vi "ETL Initialize API Connection.vi"(8 "error in (no error)":errorcluster, 11 "Base URL":string) -> (0 "error out":errorcluster, 3 "REST Client out":refnum<class "REST Client.lvclass">)   [LabVIEW 2024, in "ETL API.lvlib"]
uses:
  ETL API.lvlib
  <vilib>/addons/_JKI.lib/REST Client/classes/REST Client/REST Client.lvclass
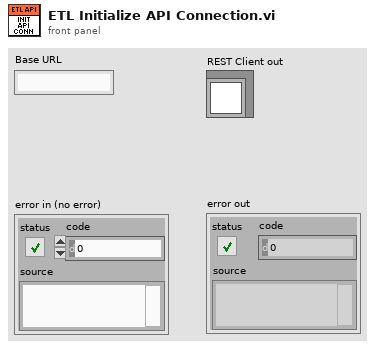
[diagram p1: front panel]
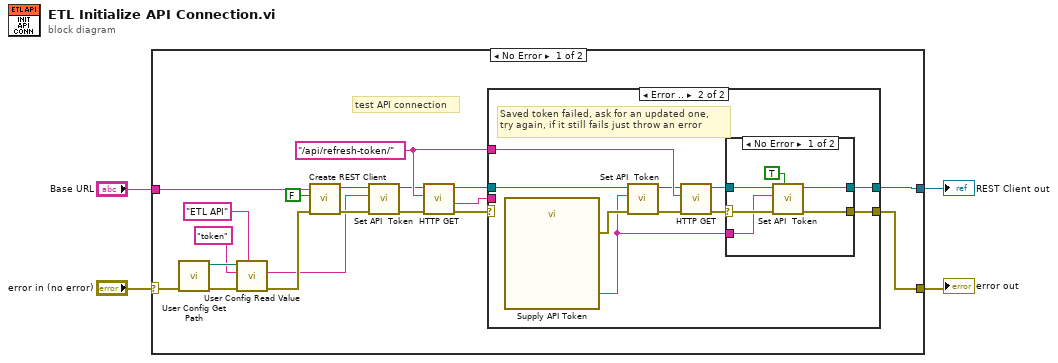
[diagram p0: block diagram]
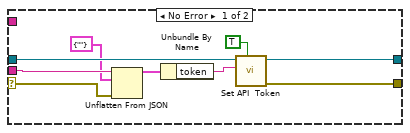
[diagram p2: hidden frame]
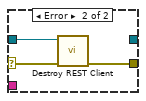
[diagram p3: hidden frame]
diagram:
  n1 = case shown="No Error" "error in (no error)" {
    selector: "error in (no error)" -> [w21 w52]
    tunnel: "Base URL" -> [w20 _]
    tunnel: [w15 w52] -> w2
    tunnel: [w16 _] -> w1
    frame No Error {
      w14 = "/api/refresh-token/" ("Path")
      # "test API connection"
      n2 = call "User Config Get Path.vi"("error in (no error)"=w21) -> ("error out"=w22:errorcluster, "INI Path"=w23:path)  [unwired: 9 in]
      n3 = call "User Config Read Value.vi"("Section"="ETL API", "error in (no error)"=w22, "Key"="token", "INI File Path"=w23) -> ("error out"=w19:errorcluster, "Value"=w10:string)  [unwired: 4 in, 2 out]
      n4 = call <vilib>:"Create REST Client.vi"("error in (no error)"=w19, "Escape URLs (true)"=FALSE, "Base URL"=w20) -> ("error out"=w11:errorcluster, "REST Client out"=w12:refnum<class "REST Client.lvclass">)  [unwired: 7 in]
      n5 = call "Set API  Token.vi"("error in (no error)"=w11, "Token"=w10, "REST Client in"=w12) -> ("error out"=w8:errorcluster, "REST Client out"=w9:refnum<class "REST Client.lvclass">)  [unwired: 7 in]
      n6 = call-dynamic "HTTP GET.vi"("error in (no error)"=w8, "Path"=w14, "REST Client in"=w9) -> ("error out"=w18:errorcluster, "Response body"=w13:string, "REST Client out"=w17:refnum<class "REST Client.lvclass">)  [unwired: 3 in, 3 out]
      n7 = case shown="Error .." w18 {
        selector: w18 -> [w31 _]
        tunnel: w17 -> [w29 w37]
        tunnel: [w28 w39] -> w16
        tunnel: [w27 w38] -> w15
        tunnel: w14 -> [_ w42]
        tunnel: w13 -> [w32 _]
        frame No Error {
          n8 = Unflatten From JSON(JSON string=w32, type and defaults=cluster{"token":string} {"token"=""}, error in (no error)=w31) -> (value=w30:cluster{"token":string})  [unwired: 4 in, 1 out]
          n9 = Unbundle By Name(w30) -> ("token"=w26:string)
          n10 = call "Set API  Token.vi"("Persist?"=TRUE, "Token"=w26, "REST Client in"=w29) -> ("error out"=w27:errorcluster, "REST Client out"=w28:refnum<class "REST Client.lvclass">)  [unwired: 7 in]
        }
        frame Error {
          # "Saved token failed, ask for an updated one, \ntry again, if it still fails just throw an error"
          n11 = call "Supply API Token"() -> ("Token"=w33:string, "error out"=w35:errorcluster)  [unwired: 17 in, 1 out]
          n12 = call "Set API  Token.vi"("error in (no error)"=w35, "Token"=w33, "REST Client in"=w37) -> ("error out"=w34:errorcluster, "REST Client out"=w36:refnum<class "REST Client.lvclass">)  [unwired: 7 in]
          n13 = call-dynamic "HTTP GET.vi"("error in (no error)"=w34, "Path"=w42, "REST Client in"=w36) -> ("error out"=w41:errorcluster, "REST Client out"=w40:refnum<class "REST Client.lvclass">)  [unwired: 3 in, 4 out]
          n14 = case shown="No Error" w41 {
            selector: w41 -> [w46 w50]
            tunnel: w40 -> [w48 w51]
            tunnel: [w47 _] -> w39
            tunnel: [w45 w49] -> w38
            tunnel: w33 -> [w44 _]
            frame No Error {
              n15 = call "Set API  Token.vi"("Persist?"=TRUE, "error in (no error)"=w46, "Token"=w44, "REST Client in"=w48) -> ("error out"=w45:errorcluster, "REST Client out"=w47:refnum<class "REST Client.lvclass">)  [unwired: 6 in]
            }
            frame Error {
              n16 = call-dynamic "Destroy REST Client.vi"("error in (no error)"=w50, "REST Client in"=w51) -> ("error out"=w49:errorcluster)  [unwired: 9 in]
            }
          }
        }
      }
    }
    frame Error {
    }
  }
  "error out" <- w2
  "REST Client out" <- w1
